vi "檢測_影像中心到邊距離.vi"(8 "error in (no error)":errorcluster, 10 "End Point":cluster{"X":i32, "Y":i32}, 11 "Image":T1) -> (0 "error out":errorcluster, 2 "Distances":sgl[](array[numeric]) format="%.4f", 3 "Image Out":T1)   [LabVIEW 2015]
uses:
  <vilib>/vision/Image Controls.llb/IMAQ Image.ctl
  <vilib>/vision/NI_Vision_Development_Module.lvlib
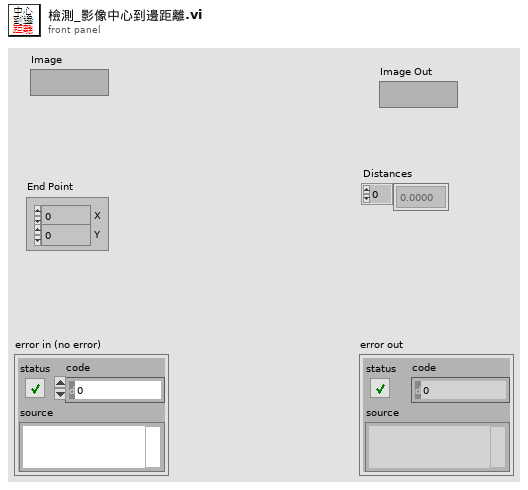
[diagram p1: front panel]
types:
  T1 = typedef "IMAQ Image.ctl" = refnum<image>
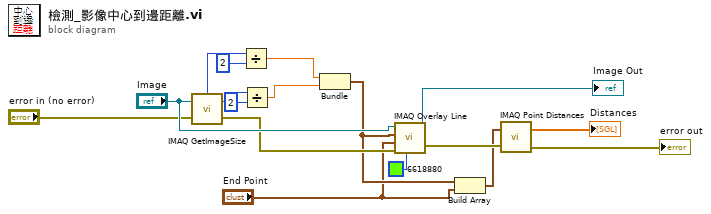
[diagram p0: block diagram]
diagram:
  n1 = call "IMAQ GetImageSize"("Image"="Image", "error in (no error)"="error in (no error)") -> ("Y Resolution"=w13:i32, "X Resolution"=w15:i32, "error out"=w11:errorcluster)  [unwired: 2 in]
  n2 = Divide(x=w15, y=2) -> (x/y=w8:dbl)
  n3 = Divide(x=w13, y=2) -> (x/y=w7:dbl)
  n4 = Bundle(w8, w7) -> (w5:cluster{dbl, dbl})  [unwired: 1 in]
  n5 = call "IMAQ Overlay Line"("Color"=u32 6618880, "error in (no error)"=w11, "End Point"="End Point", "Start Point"=w5, "Image"="Image") -> ("error out"=w17:errorcluster, "Image Out"=→"Image Out":T1)  [unwired: 5 in]
  n6 = Build Array(w5, "End Point") -> (w3:cluster{"X":dbl, "Y":dbl}[])
  n7 = call "IMAQ Point Distances"("Points"=w3, "error in (no error)"=w17) -> ("Distances"=→"Distances":sgl[], "error out"=→"error out":errorcluster)  [unwired: 3 in]
